vi "Serial Interface.vi"(1 "UART Inputs":T2={"Tx Data"=[0, 0, 0, 0, 0, 0, 0, 0, 0, 0], "Transmit"=FALSE, "Receive"=FALSE, "Byte Mode"=TRUE, "Set Baud Rate"=FALSE, "Baud Rate"=0} {"Baud Rate" format="%02x"; "Tx Data" format="%02x"}) -> (0 "UART Outputs":T1 {"Rx Data" format="%02x"})   [LabVIEW 2014]
uses:
  <vilib>/rvi/eio/common/nirviEmuTemplateMethod_errors.vi
  <vilib>/eio/EIONode/EIONode.xnode
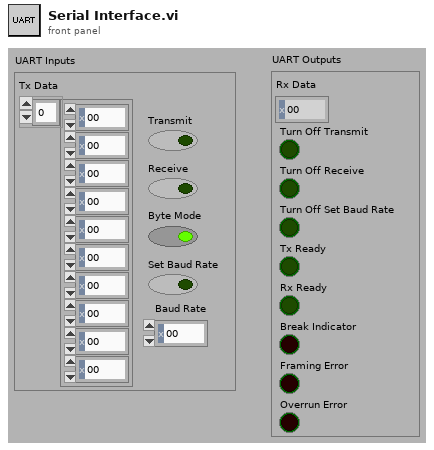
[diagram p1: front panel]
types:
  T1 = cluster{"Rx Data":u8, "Turn Off Transmit":bool, "Turn Off Receive":bool, "Turn Off Set Baud Rate":bool, "Tx Ready":bool, "Rx Ready":bool, "Break Indicator":bool, "Framing Error":bool, "Overrun Error":bool}
  T2 = cluster{"Tx Data":u8[], "Transmit":bool, "Receive":bool, "Byte Mode":bool, "Set Baud Rate":bool, "Baud Rate":u8}
  T3 = enum16{"Idle", "Wait For Ready", "Send Byte", "Check If Done"}
  T4 = enum16{"Idle", "Assert Read", "Latch Data", "Done"}
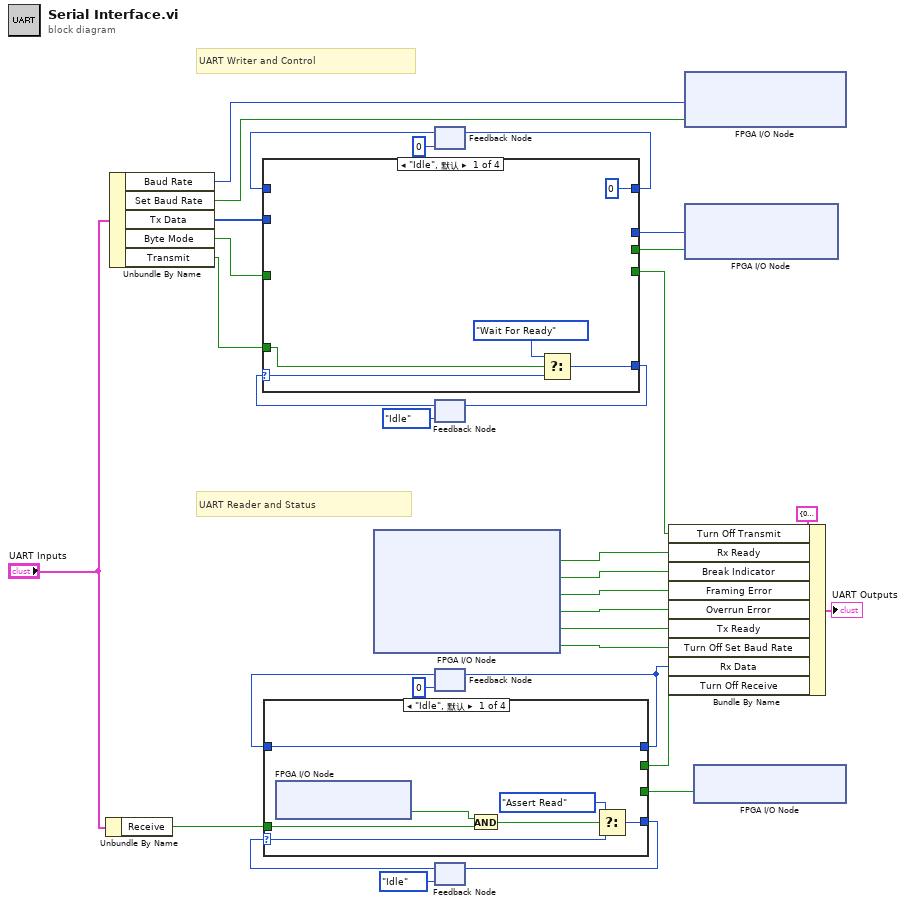
[diagram p0: block diagram]
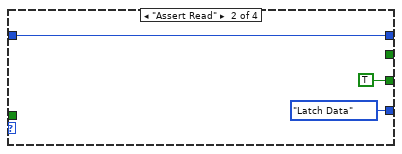
[diagram p2: hidden frame]
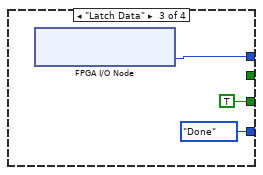
[diagram p3: hidden frame]
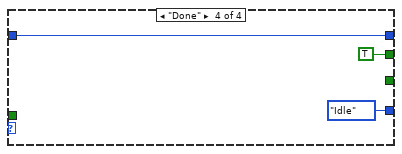
[diagram p4: hidden frame]
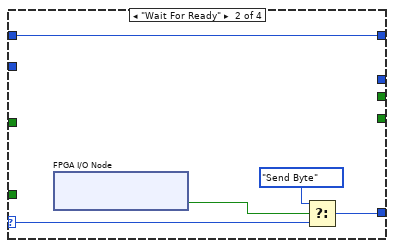
[diagram p5: hidden frame]
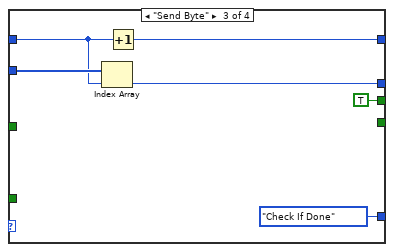
[diagram p6: hidden frame]
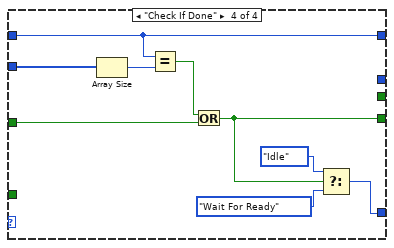
[diagram p7: hidden frame]
diagram:
  # "UART Writer and Control"
  # "UART Reader and Status"
  n1 = Unbundle By Name("UART Inputs") -> ("Receive"=w10:bool)
  n2 = Unbundle By Name("UART Inputs") -> ("Baud Rate"=w11:u8, "Set Baud Rate"=w9:bool, "Tx Data"=w14:u8[], "Byte Mode"=w5:bool, "Transmit"=w6:bool)
  n3 = xnode "FPGA I/O Node"() -> ("UART RX Ready"=w12:bool, "UART Break Indicator"=w21:bool, "UART Framing Error"=w20:bool, "UART RX Overrun Error"=w19:bool, "UART TX Ready"=w18:bool, "UART Set Baud Rate Ack"=w17:bool)  [unwired: 6 in, 6 out]
  n4 = feedback #1(u8 0) -> (w30:u8)
  n5 = feedback #2(T3."Idle") -> (w3:T3)
  n6 = case shown="\"Idle\", 默认" w3 {
    selector: w3 -> [w34 w40 _ _]
    tunnel: w6 -> [w33 _ _ _]
    tunnel: [w35 w41 T3."Check If Done" w50] -> w2
    tunnel: [_ _ TRUE _] -> w28
    tunnel: w14 -> [_ _ w47 w57]
    tunnel: w30 -> [_ w38 w46 w55]
    tunnel: [u8 0 w38 w45 w55] -> w29
    tunnel: [_ _ w44 _] -> w32
    tunnel: w5 -> [_ _ _ w53]
    tunnel: [_ _ _ w49] -> w1
    frame "Idle", Default {
      n7 = Select(t=T3."Wait For Ready", s=w33, f=w34) -> (s? t:f=w35:T3)
    }
    frame "Wait For Ready" {
      n8 = xnode "FPGA I/O Node"() -> ("UART TX Ready"=w39:bool)  [unwired: 1 in, 1 out]
      n9 = Select(t=T3."Send Byte", s=w39, f=w40) -> (s? t:f=w41:T3)
    }
    frame "Send Byte" {
      n10 = Index Array(array=w47, index=w46) -> (element=w44:u8)
      n11 = Increment(x=w46) -> (x+1=w45:u8)
    }
    frame "Check If Done" {
      n12 = Array Size(array=w57) -> (size(s)=w56:i32)
      n13 = Equal?(x=w55, y=w56) -> (x = y?=w54:bool)
      n14 = Or(x=w54, y=w53) -> (x .or. y?=w49:bool)
      n15 = Select(t=T3."Idle", s=w49, f=T3."Wait For Ready") -> (s? t:f=w50:T3)
    }
  }
  n16 = feedback-in #1(w29) -> ()
  n17 = feedback-in #2(w2) -> ()
  n18 = feedback #3(u8 0 ("IO Module\\rUartDataOut")) -> (w22:u8)
  n19 = feedback #4(T4."Idle") -> (w25:T4)
  n20 = case shown="\"Idle\", 默认" w25 {
    selector: w25 -> [w63 _ _ _]
    tunnel: w10 -> [w59 _ _ _]
    tunnel: [w64 T4."Latch Data" ("t") T4."Done" ("t") T4."Idle" ("t")] -> w24
    tunnel: [_ TRUE TRUE _] -> w27
    tunnel: [w61 w65 w68 w72] -> w15
    tunnel: w22 -> [w61 w65 _ w72]
    tunnel: [_ _ _ TRUE] -> w16
    frame "Idle", Default {
      n21 = xnode "FPGA I/O Node"() -> ("UART RX Ready"=w58:bool)  [unwired: 1 in, 1 out]
      n22 = And(x=w58, y=w59) -> (x .and. y?=w60:bool)
      n23 = Select(t=T4."Assert Read", s=w60, f=w63) -> (s? t:f=w64:T4)
    }
    frame "Assert Read" {
    }
    frame "Latch Data" {
      n24 = xnode "FPGA I/O Node"() -> ("UART Read Data"=w68:u8)  [unwired: 1 in, 1 out]
    }
    frame "Done" {
    }
  }
  n25 = feedback-in #3(w15) -> ()
  n26 = feedback-in #4(w24) -> ()
  n27 = Bundle By Name(cluster=T1 {"Rx Data"=0, "Turn Off Transmit"=FALSE, "Turn Off Receive"=FALSE, "Turn Off Set Baud Rate"=FALSE, "Tx Ready"=FALSE, "Rx Ready"=FALSE, "Break Indicator"=FALSE, "Framing Error"=FALSE, "Overrun Error"=FALSE} ("UART Outputs"), "Turn Off Transmit"=w1, "Rx Ready"=w12, "Break Indicator"=w21, "Framing Error"=w20, "Overrun Error"=w19, "Tx Ready"=w18, "Turn Off Set Baud Rate"=w17, "Rx Data"=w15, "Turn Off Receive"=w16) -> (→"UART Outputs":T1)
  n28 = xnode "FPGA I/O Node"("UART Baud Rate In"=w11, "UART Set Baud Rate"=w9) -> ()  [unwired: 2 in, 2 out]
  n29 = xnode "FPGA I/O Node"("UART Write Data"=w32, "UART Write Enable"=w28) -> ()  [unwired: 2 in, 2 out]
  n30 = xnode "FPGA I/O Node"("UART Read Enable"=w27) -> ()  [unwired: 1 in, 1 out]
